vi "Log Data.vi"(8 "error in (no error)":errorcluster, 11 "Bioreactor in":refnum<class "Bioreactor.lvclass">) -> (0 "error out":errorcluster, 3 "Bioreactor out":refnum<class "Bioreactor.lvclass">)   [LabVIEW 2013, in "Bioreactor.lvlib" / "Bioreactor.lvclass"]
uses:
  Bioreactor.lvclass
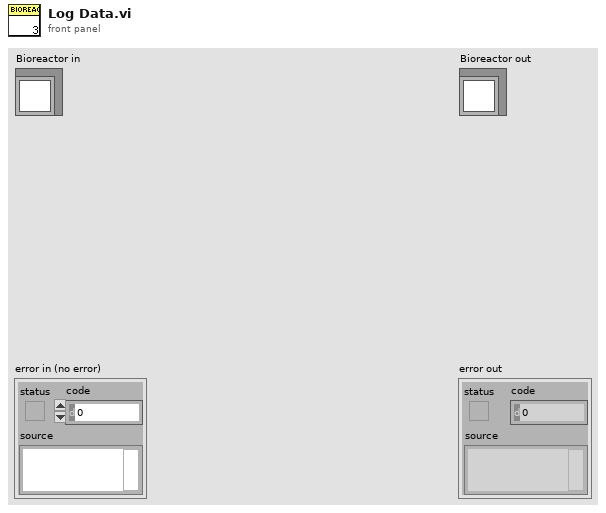
[diagram p1: front panel]
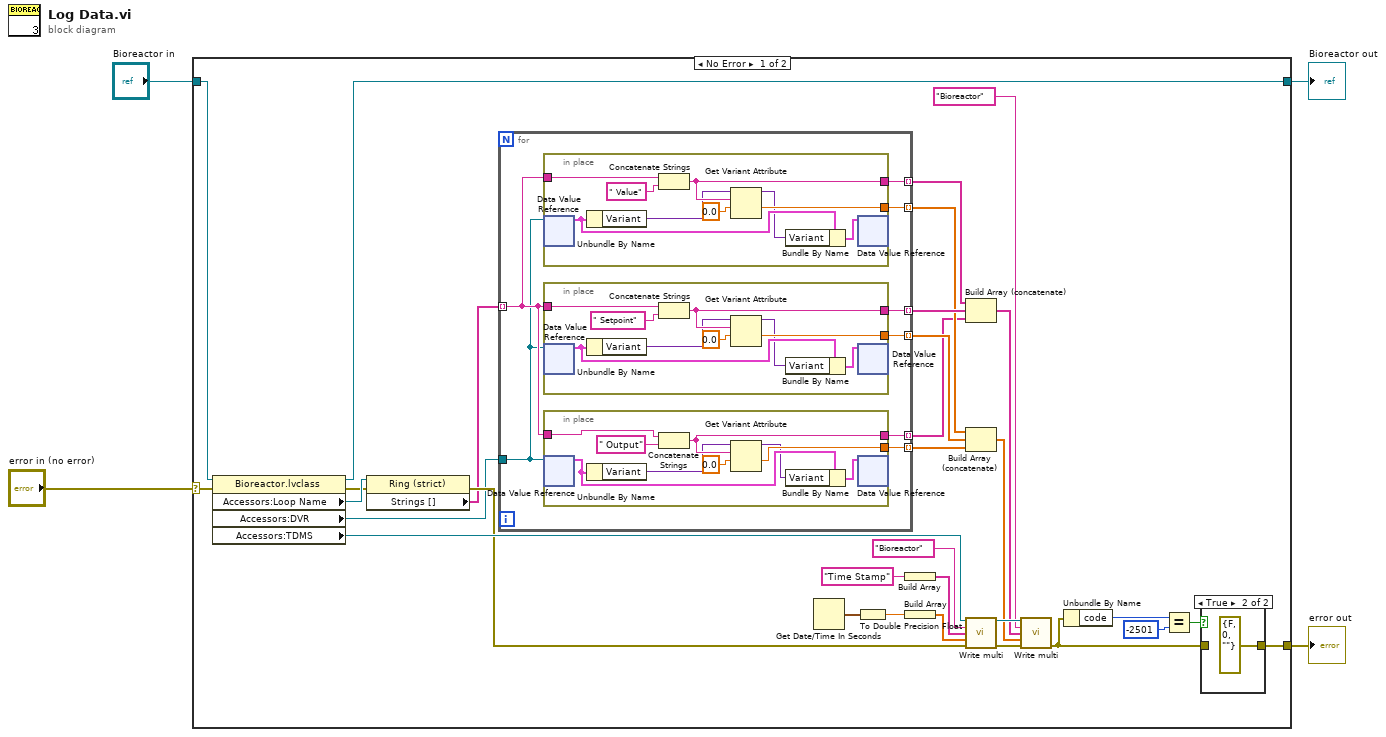
[diagram p0: block diagram]
diagram:
  n1 = case shown="No Error" "error in (no error)" {
    selector: "error in (no error)" -> [w34 w74]
    tunnel: [w32 w74] -> w3
    tunnel: [w33 w73] -> w1
    tunnel: "Bioreactor in" -> [w35 w73]
    frame No Error {
      n2 = property class="Bioreactor.lvclass"(reference=w35, error in=w34) -> (reference out=w33:refnum<class "Bioreactor.lvclass">, error out=w17:errorcluster, "Accessors:Loop Name"=w18:refnum<vi>, "Accessors:DVR"=w11:refnum<data-value>, "Accessors:TDMS"=w19:refnum<k34>)
      n3 = property class="Ring (strict)"(reference=w18, error in=w17) -> (error out=w16:errorcluster, "Strings []"=w12:string[])  [unwired: 1 out]
      n4 = for {
        tunnel: w12 -> [w43] mode=indexing
        tunnel: w11 -> [w42]
        tunnel: [w41] -> w10 mode=indexing
        tunnel: [w40] -> w9 mode=indexing
        tunnel: [w39] -> w8 mode=indexing
        tunnel: [w38] -> w7 mode=indexing
        tunnel: [w37] -> w6 mode=indexing
        tunnel: [w36] -> w5 mode=indexing
        n5 = in-place {
          in-place-border: w43 -> [w52]
          in-place-border: [w49] -> w39
          in-place-border: [w48] -> w41
          n6 = in-place-dvr #1(w42) -> (w46:cluster{"Array":string[], "Variant":variant})  [unwired: 1 out]
          n7 = Unbundle By Name(w46) -> ("Variant"=w45:variant)
          n8 = Concatenate Strings(w52, " Value" ("string")) -> (w48:string)
          n9 = Get Variant Attribute(Variant=w45, name=w48, default value (empty Variant)=0.0 ("Value")) -> (duplicate Variant=w44:variant, value=w49:dbl)  [unwired: 1 in, 2 out]
          n10 = Bundle By Name(cluster=w46, "Variant"=w44) -> (w47:cluster{"Array":string[], "Variant":variant})
          n11 = in-place-dvr #1(w47) -> ()  [unwired: 2 out]
        }
        n12 = in-place {
          in-place-border: w43 -> [w70]
          in-place-border: [w69] -> w38
          in-place-border: [w66] -> w40
          n13 = in-place-dvr #2(w42) -> (w63:cluster{"Array":string[], "Variant":variant})  [unwired: 1 out]
          n14 = Unbundle By Name(w63) -> ("Variant"=w64:variant)
          n15 = Concatenate Strings(w70, " Setpoint" ("string")) -> (w66:string)
          n16 = Get Variant Attribute(Variant=w64, name=w66, default value (empty Variant)=0.0 ("Value")) -> (duplicate Variant=w62:variant, value=w69:dbl)  [unwired: 1 in, 2 out]
          n17 = Bundle By Name(cluster=w63, "Variant"=w62) -> (w65:cluster{"Array":string[], "Variant":variant})
          n18 = in-place-dvr #2(w65) -> ()  [unwired: 2 out]
        }
        n19 = in-place {
          in-place-border: w43 -> [w61]
          in-place-border: [w60] -> w36
          in-place-border: [w57] -> w37
          n20 = in-place-dvr #3(w42) -> (w54:cluster{"Array":string[], "Variant":variant})  [unwired: 1 out]
          n21 = Unbundle By Name(w54) -> ("Variant"=w55:variant)
          n22 = Concatenate Strings(w61, " Output" ("string")) -> (w57:string)
          n23 = Get Variant Attribute(Variant=w55, name=w57, default value (empty Variant)=0.0 ("Value")) -> (duplicate Variant=w53:variant, value=w60:dbl)  [unwired: 1 in, 2 out]
          n24 = Bundle By Name(cluster=w54, "Variant"=w53) -> (w56:cluster{"Array":string[], "Variant":variant})
          n25 = in-place-dvr #3(w56) -> ()  [unwired: 2 out]
        }
      }
      n26 = Get Date/Time In Seconds() -> (seconds since 1Jan1904=w31:timestamp)
      n27 = To Double Precision Float(number=w31) -> (double precision float=w28:dbl)
      n28 = Build Array("Time Stamp" ("Channel")) -> (w29:string[])
      n29 = Build Array(w28) -> (w27:dbl[])
      n30 = Build Array (concatenate)(w10, w9, w6) -> (w15:string[])
      n31 = Build Array (concatenate)(w8, w7, w5) -> (w14:dbl[])
      n32 = call "Write multi.vi"("tdms file in"=w19, "group"="Bioreactor", "Channel"=w29, "Data"=w27, "error in (no error)"=w16) -> ("tdms file out"=w25:refnum<k34>, "error out"=w26:errorcluster)  [unwired: 7 in, 2 out]
      n33 = call "Write multi.vi"("tdms file in"=w25, "group"="Bioreactor", "Channel"=w15, "Data"=w14, "error in (no error)"=w26) -> ("error out"=w20:errorcluster)  [unwired: 7 in, 3 out]
      n34 = Unbundle By Name(w20) -> ("code"=w23:i32)
      n35 = Equal?(x=w23, y=-2501) -> (x = y?=w21:bool)
      n36 = case shown="True" w21 {
        tunnel: w20 -> [w71 _]
        tunnel: [w71 errorcluster {"status"=FALSE, "code"=0, "source"=""} ("error constant")] -> w32
        frame False {
        }
        frame True {
        }
      }
    }
    frame Error {
    }
  }
  "error out" <- w3
  "Bioreactor out" <- w1
